vi "Create Audio Analyzer Display Objects.vi"(8 "Error In":errorcluster, 11 "Display Manager In":refnum<class "Display Manager.lvclass">) -> (0 "Error Out":errorcluster, 3 "Display Manager Out":refnum<class "Display Manager.lvclass">)   [LabVIEW 2019, in "Display Manager.lvclass"]
uses:
  Display Manager.lvclass
  <vilib>/Memosfet/myRIO-Neopixel/RT/Display Utilities/Public/Controls/2D Coordinates.ctl
  <vilib>/Memosfet/myRIO-Neopixel/RT/Graph/Graph.lvclass
  C:/Program Files (x86)/National Instruments/LabVIEW 2019/vi.lib/Memosfet/myRIO-Neopixel/RT/Display Element/Display Element.lvclass
  <vilib>/Memosfet/myRIO-Neopixel/RT/Graph/Public/Controls/Fill To.ctl
  <vilib>/Memosfet/myRIO-Neopixel/RT/Graph/Public/Controls/Range.ctl
  Accessors/Display/Get Display.vi
  <vilib>/Memosfet/myRIO-Neopixel/RT/Display/Display.lvclass
  <vilib>/Memosfet/myRIO-Neopixel/RT/Display Utilities/Display Utilities.lvlib
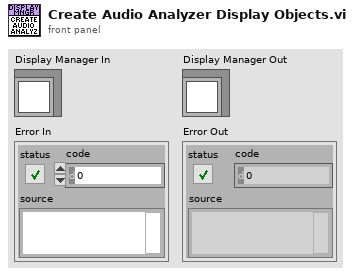
[diagram p1: front panel]
types:
  T1 = typedef "Graph.lvclass/Range.ctl" = cluster{"Maximum":dbl, "Minimum":dbl}
  T2 = typedef "Graph.lvclass/Fill To.ctl" = enum16{"None", "Inf", "-Inf"}
  T3 = typedef "Display Utilities.lvlib/2D Coordinates.ctl" = cluster{"X":i32, "Y":i32}
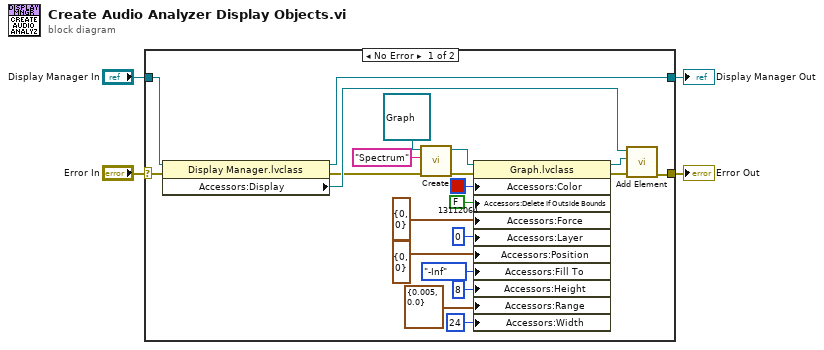
[diagram p0: block diagram]
diagram:
  n1 = case shown="No Error" "Error In" {
    selector: "Error In" -> [w19 w27]
    tunnel: [w10 w27] -> w3
    tunnel: "Display Manager In" -> [w20 w26]
    tunnel: [w15 w26] -> w1
    frame No Error {
      n2 = property class="Display Manager.lvclass"(reference=w20, error in=w19) -> (reference out=w15:refnum<class "Display Manager.lvclass">, error out=w17:errorcluster, "Accessors:Display"=w18:refnum<class "Display.lvclass">)
      n3 = call-dynamic "Create.vi"("Error In"=w17, "Tag"="Spectrum", "Graph In"=refnum<class "Graph.lvclass"> refnum) -> ("Error Out"=w14:errorcluster, "Graph Out"=w13:refnum<class "Graph.lvclass">)  [unwired: 7 in]
      n4 = property class="Graph.lvclass"(reference=w13, error in=w14, "Accessors:Color"=u32 13112064 ("Color"), "Accessors:Delete If Outside Bounds"=FALSE ("Delete If Outside Bounds"), "Accessors:Force"=T3 {"X"=0, "Y"=0} ("Force"), "Accessors:Layer"=u32 0 ("Layer"), "Accessors:Position"=T3 {"X"=0, "Y"=0} ("Position"), "Accessors:Fill To"=Fill_To."-Inf" ("Fill To"), "Accessors:Height"=u32 8 ("Height"), "Accessors:Range"=T1 {"Maximum"=0.005, "Minimum"=0.0} ("Range"), "Accessors:Width"=u32 24 ("Width")) -> (reference out=w11:refnum<class "Graph.lvclass">, error out=w12:errorcluster)
      n5 = call <vilib>:"Add Element.vi"("Error In"=w12, "New Element"=w11, "Display In"=w18) -> ("Error Out"=w10:errorcluster)  [unwired: 7 in, 1 out]
    }
    frame Error {
    }
  }
  "Display Manager Out" <- w1
  "Error Out" <- w3
